vi "Calculate Measurements.vi"(8 "error in (no error)":errorcluster, 11 "Program Data":T2={"Measurements"={"Channel 0"="", "RMS 0"="", "Vp-p 0"="", "Freq 0"="", "Channel 1"="", "RMS 1"="", "Vp-p 1"="", "Freq 1"="", "Cursors"="", "C1"="", "C2"="", "dT"=""}, "C1"={"Name"="", "X"=0.0, "Y"=0.0}, "C2"={"Name"="", "X"=0.0, "Y"=0.0}, "Com"={"Connection Info"={"connection ID"=refnum, "meta data"=[]}, "Connected?"=FALSE, "IP"=""}, "Continuous?"=FALSE, "Scope Data"={"AI0"=[], "AI1"=[]}, "Wave Parameters"={"Frequency (Hz)"=0.0, "Phase offset (deg)"=0.0, "Vpeak (V)"=0.0, "Offset (V)"=0.0, "Waveform"=enum."Sine", "Channel"=enum."CH0"}, "Acquire?"=FALSE, "Measure Ref"=refnum, "CH0"={"Channel"=enum."AI 0", "Enable"=TRUE, "Volts/Div"=5, "Vertical Position (Div)"=0.0}, "CH1"={"Channel"=enum."AI 1", "Enable"=FALSE, "Volts/Div"=5, "Vertical Position (Div)"=0.0}, "CH0 Params"={"V/Div"=0.5, "Units"="V"}, "CH1 Params"={"V/Div"=0.5, "Units"="V"}, "Time"={"Time/Div"=0.0}, "dT"=0.0, "FGen"={"Offset (V)"=0.0, "Enable Sweep"=FALSE, "Start Frequency (Hz)"=0.0, "Stop Frequency (Hz)"=0.0, "Step (Hz)"=0.0, "Step Interval (ms)"=0.0, "Current Freq (Hz)"=0.0, "Run"=FALSE}} {"Time"."Time/Div" min=0.0 max=16.0 step=1.0 scale=0.0..12.0; "CH1"."Vertical Position (Div)" min=-5.0 max=5.0 step=0.1 scale=-5.0..5.0; "CH1"."Volts/Div" min=0 max=8 step=1 scale=0.0..8.0; "CH0"."Vertical Position (Div)" min=-5.0 max=5.0 step=0.1 scale=-5.0..5.0; "CH0"."Volts/Div" min=0 max=8 step=1 scale=0.0..8.0; "Wave Parameters"."Phase offset (deg)" format="%#_6p"; "Wave Parameters"."Frequency (Hz)" format="%#_6p"}) -> (0 "error out":errorcluster, 3 "Program Data Out":T2={"Measurements"={"Channel 0"="", "RMS 0"="", "Vp-p 0"="", "Freq 0"="", "Channel 1"="", "RMS 1"="", "Vp-p 1"="", "Freq 1"="", "Cursors"="", "C1"="", "C2"="", "dT"=""}, "C1"={"Name"="", "X"=0.0, "Y"=0.0}, "C2"={"Name"="", "X"=0.0, "Y"=0.0}, "Com"={"Connection Info"={"connection ID"=refnum, "meta data"=[]}, "Connected?"=FALSE, "IP"=""}, "Continuous?"=FALSE, "Scope Data"={"AI0"=[], "AI1"=[]}, "Wave Parameters"={"Frequency (Hz)"=0.0, "Phase offset (deg)"=0.0, "Vpeak (V)"=0.0, "Offset (V)"=0.0, "Waveform"=enum."Sine", "Channel"=enum."CH0"}, "Acquire?"=FALSE, "Measure Ref"=refnum, "CH0"={"Channel"=enum."AI 0", "Enable"=TRUE, "Volts/Div"=5, "Vertical Position (Div)"=0.0}, "CH1"={"Channel"=enum."AI 1", "Enable"=FALSE, "Volts/Div"=5, "Vertical Position (Div)"=0.0}, "CH0 Params"={"V/Div"=0.5, "Units"="V"}, "CH1 Params"={"V/Div"=0.5, "Units"="V"}, "Time"={"Time/Div"=0.0}, "dT"=0.0, "FGen"={"Offset (V)"=0.0, "Enable Sweep"=FALSE, "Start Frequency (Hz)"=0.0, "Stop Frequency (Hz)"=0.0, "Step (Hz)"=0.0, "Step Interval (ms)"=0.0, "Current Freq (Hz)"=0.0, "Run"=FALSE}} {"Time"."Time/Div" min=0.0 max=16.0 step=1.0 scale=0.0..12.0; "CH1"."Vertical Position (Div)" min=-5.0 max=5.0 step=0.1 scale=-5.0..5.0; "CH1"."Volts/Div" min=0 max=8 step=1 scale=0.0..8.0; "CH0"."Vertical Position (Div)" min=-5.0 max=5.0 step=0.1 scale=-5.0..5.0; "CH0"."Volts/Div" min=0 max=8 step=1 scale=0.0..8.0; "Wave Parameters"."Phase offset (deg)" format="%#_6p"; "Wave Parameters"."Frequency (Hz)" format="%#_6p"})   [LabVIEW 2021]
uses:
  Controls/Program Data.ctl
  Controls/Measurements.ctl
  Controls/Channel Measurement String Control.ctl
  Controls/Cursor Info.ctl
  Controls/Communication Cluster.ctl
  <vilib>/NI/STM/TCP/TCP Connection Info.ctl
  <vilib>/NI/STM/SubVIs/MetaDataElement.ctl
  Communication/Scope Data.ctl
  Program Files (x86)/National Instruments/LabVIEW 2021/ProjectTemplates/Source/myRIO/Oscilloscope/myRIO v1.1/Real-Time/Controls/Wave Parameters.ctl
  Program Files (x86)/National Instruments/LabVIEW 2021/ProjectTemplates/Source/myRIO/Oscilloscope/myRIO v1.1/Real-Time/Controls/Waveform Enum.ctl
  Program Files (x86)/National Instruments/LabVIEW 2021/ProjectTemplates/Source/myRIO/Oscilloscope/myRIO v1.1/Real-Time/Controls/Channel Selector.ctl
  Controls/Channel Settings.ctl
  Controls/Analog Input Selector.ctl
  Controls/Knob.ctl
  Controls/Vertical Position.ctl
  Controls/Channel Parameters.ctl
  Controls/Time Selector.ctl
  Controls/Time Knob.ctl
  Controls/FGen Desktop Configuration.ctl
  <vilib>/measure/matone.llb/Extract Single Tone Information 1 Chan.vi
  <vilib>/measure/madcrms.llb/Basic Averaged DC-RMS for 1 Chan.vi
  <vilib>/measure/NI_MAPro.lvlib
  <vilib>/NI/STM/NI STM.lvlib
panel:
  in  "advanced search":T1={"approx freq. (optional)"=-1.0, "search (+/- % of Fsampl.)"=5.0} {"search (+/- % of Fsampl.)" format="%0.2p"; "approx freq. (optional)" format="%0.2p"}
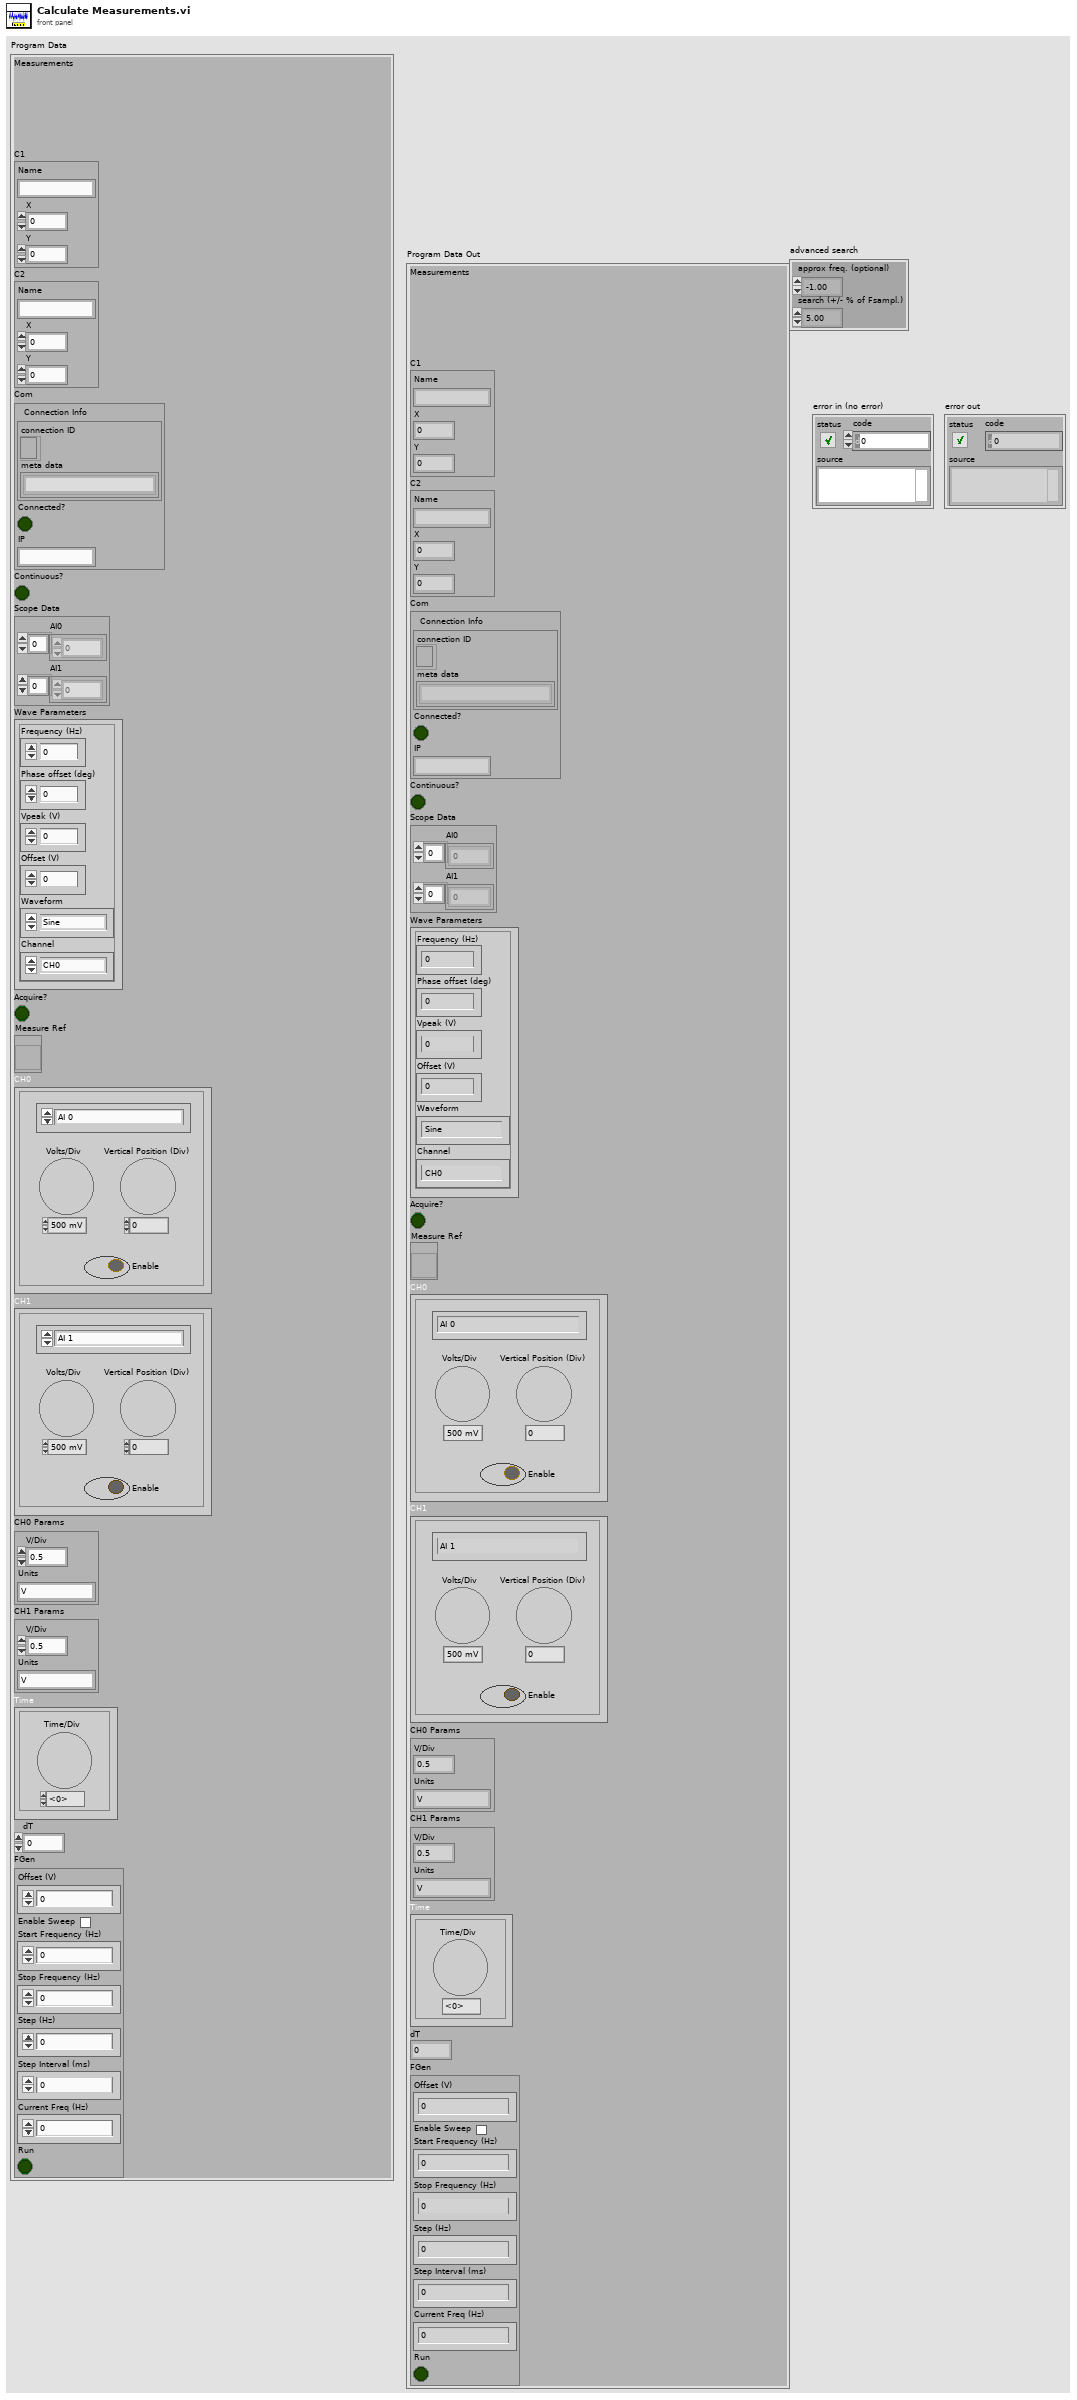
[diagram p1: front panel]
types:
  T1 = cluster{"approx freq. (optional)":dbl, "search (+/- % of Fsampl.)":dbl}
  T2 = typedef "Program Data.ctl" = cluster{"Measurements":T3, "C1":T5, "C2":T5, "Com":T6, "Continuous?":bool, "Scope Data":T9, "Wave Parameters":T10, "Acquire?":bool, "Measure Ref":refnum<vi>, "CH0":T13, "CH1":T13, "CH0 Params":T17, "CH1 Params":T17, "Time":T18, "dT":dbl, "FGen":T20}
  T3 = typedef "Measurements.ctl" = cluster{"Channel 0":T4, "RMS 0":T4, "Vp-p 0":T4, "Freq 0":T4, "Channel 1":T4, "RMS 1":T4, "Vp-p 1":T4, "Freq 1":T4, "Cursors":T4, "C1":T4, "C2":T4, "dT":T4}
  T4 = typedef "Channel Measurement String Control.ctl" = string
  T5 = typedef "Cursor Info.ctl" = cluster{"Name":string, "X":dbl, "Y":dbl}
  T6 = typedef "Communication Cluster.ctl" = cluster{"Connection Info":T7, "Connected?":bool, "IP":string}
  T7 = typedef "NI STM.lvlib/TCP Connection Info.ctl" = cluster{"connection ID":refnum<k5>, "meta data":T8[]}
  T8 = typedef "NI STM.lvlib/MetaDataElement.ctl" = string
  T9 = typedef "Scope Data.ctl" = cluster{"AI0":dbl[], "AI1":dbl[]}
  T10 = typedef "Wave Parameters.ctl" = cluster{"Frequency (Hz)":dbl, "Phase offset (deg)":dbl, "Vpeak (V)":dbl, "Offset (V)":dbl, "Waveform":T11, "Channel":T12}
  T11 = typedef "Waveform Enum.ctl" = enum16{"Sine", "Square"}
  T12 = typedef "Channel Selector.ctl" = enum16{"CH0", "CH1"}
  T13 = typedef "Channel Settings.ctl" = cluster{"Channel":T14, "Enable":bool, "Volts/Div":T15, "Vertical Position (Div)":T16}
  T14 = typedef "Analog Input Selector.ctl" = enum16{"AI 0", "AI 1"}
  T15 = typedef "Knob.ctl" = i32
  T16 = typedef "Vertical Position.ctl" = dbl
  T17 = typedef "Channel Parameters.ctl" = cluster{"V/Div":dbl, "Units":string}
  T18 = typedef "Time Selector.ctl" = cluster{"Time/Div":T19}
  T19 = typedef "Time Knob.ctl" = dbl
  T20 = typedef "FGen Desktop Configuration.ctl" = cluster{"Offset (V)":dbl, "Enable Sweep":bool, "Start Frequency (Hz)":dbl, "Stop Frequency (Hz)":dbl, "Step (Hz)":dbl, "Step Interval (ms)":dbl, "Current Freq (Hz)":dbl, "Run":bool}
  T21 = enum32{"none", "input signal", "detected signal", "residual signal"}
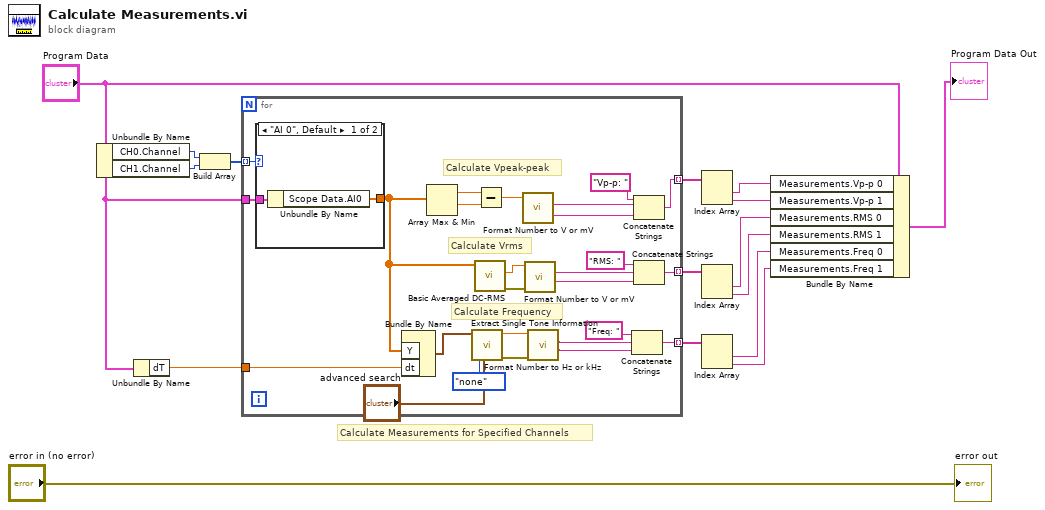
[diagram p0: block diagram]
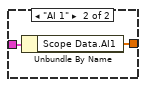
[diagram p2: hidden frame]
diagram:
  # "Calculate Measurements for Specified Channels"
  n1 = Unbundle By Name("Program Data") -> ("CH0.Channel"=w16:T14, "CH1.Channel"=w15:T14)
  n2 = Unbundle By Name("Program Data") -> ("dT"=w1:dbl)
  n3 = Build Array(w16, w15) -> (w14:T14[])
  n4 = for {
    tunnel: [w42] -> w13 mode=indexing
    tunnel: w14 -> [w23] mode=indexing
    tunnel: "Program Data" -> [w41]
    tunnel: [w40] -> w9 mode=indexing
    tunnel: [w39] -> w6 mode=indexing
    tunnel: w1 -> [w17]
    # "Calculate Frequency"
    # "Calculate Vrms"
    # "Calculate Vpeak-peak"
    n5 = case shown="\"AI 0\", Default" w23 {
      tunnel: w41 -> [w44 w46]
      tunnel: [w43 w45] -> w18
      frame "AI 0", Default {
        n6 = Unbundle By Name(w44) -> ("Scope Data.AI0"=w43:dbl[])
      }
      frame "AI 1" {
        n7 = Unbundle By Name(w46) -> ("Scope Data.AI1"=w45:dbl[])
      }
    }
    n8 = Bundle By Name("Y"=w18, "dt"=w17) -> (w20:waveform(dbl))  [unwired: 1 in]
    n9 = Array Max & Min(array=w18) -> (max value=w35:dbl, min value=w36:dbl)  [unwired: 2 out]
    n10 = call-poly <vilib>:"Extract Single Tone Information.vi"("advanced search"="advanced search", "export mode"=T21."none", "time signal in"=w20) -> ("error out"=w24:errorcluster, "detected frequency"=w21:dbl)  [unwired: 3 in, 4 out]
    n11 = call-poly <vilib>:"Basic Averaged DC-RMS.vi"("signal in"=w18) -> ("error out"=w31:errorcluster, "RMS value"=w30:dbl)  [unwired: 7 in, 2 out]
    n12 = Subtract(x=w35, y=w36) -> (x-y=w37:dbl)
    n13 = call "Format Number to V or mV.vi"("Value"=w37) -> ("Units"=w33:string, "Value Out"=w34:string)  [unwired: 7 in, 2 out]
    n14 = call "Format Number to V or mV.vi"("error in (no error)"=w31, "Value"=w30) -> ("Units"=w28:string, "Value Out"=w29:string)  [unwired: 6 in, 2 out]
    n15 = call "Format Number to Hz or kHz.vi"("error in (no error)"=w24, "Value"=w21) -> ("Units"=w25:string, "Value Out"=w26:string)  [unwired: 6 in, 2 out]
    n16 = Concatenate Strings("Freq: " ("string"), w26, w25) -> (w39:string)
    n17 = Concatenate Strings("Vp-p: " ("string"), w34, w33) -> (w42:string)
    n18 = Concatenate Strings("RMS: " ("string"), w29, w28) -> (w40:string)
  }
  n19 = Index Array(array=w13) -> (element #1=w12:string, element #2=w11:string)  [unwired: 2 in]
  n20 = Index Array(array=w9) -> (element #1=w8:string, element #2=w7:string)  [unwired: 2 in]
  n21 = Index Array(array=w6) -> (element #1=w5:string, element #2=w4:string)  [unwired: 2 in]
  n22 = Bundle By Name(cluster="Program Data", "Measurements.Vp-p 0"=w12, "Measurements.Vp-p 1"=w11, "Measurements.RMS 0"=w8, "Measurements.RMS 1"=w7, "Measurements.Freq 0"=w5, "Measurements.Freq 1"=w4) -> (→"Program Data Out":T2)
  "error out" <- "error in (no error)"
